vi "ADC_clock.vi"(6 "phase":u8, 10 "iterations per cycle":u8=4, 11 "counter in":u8) -> (3 "counter out":u8)   [LabVIEW 2011]
uses:
  <vilib>/rvi/eio/common/nirviEmuTemplateMethod_errors.vi
  <vilib>/eio/EIONode/EIONode.xnode
panel:
  out "clock signal high?":bool
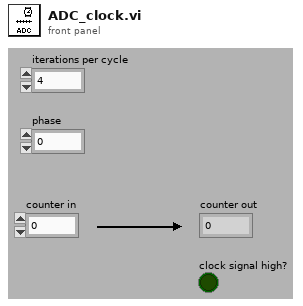
[diagram p1: front panel]
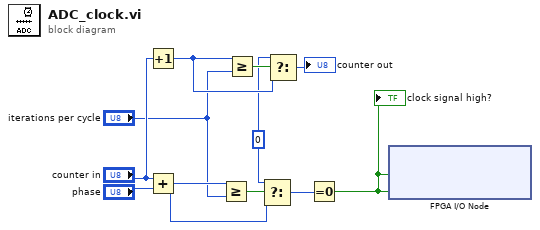
[diagram p0: block diagram]
diagram:
  w1 = u8 0
  n1 = Increment(x="counter in") -> (x+1=w8:u8)
  n2 = Add(x="counter in", y="phase") -> (x+y=w5:u8)
  n3 = Greater Or Equal?(x=w5, y="iterations per cycle") -> (x >= y?=w6:bool)
  n4 = Greater Or Equal?(x=w8, y="iterations per cycle") -> (x >= y?=w11:bool)
  n5 = Select(t=w1, s=w6, f=w5) -> (s? t:f=w4:u8)
  n6 = Select(t=w1, s=w11, f=w8) -> (s? t:f=→"counter out":u8)
  n7 = Equal To 0?(x=w4) -> (x = 0?=w3:bool)
  "clock signal high?" <- w3
  n8 = xnode "FPGA I/O Node"("Connector0/DIO15"=w3, "Connector1/DIO15"=w3) -> ()  [unwired: 2 in, 2 out]
